vi "Set HW ID.vi"(8 "error in (no error)":errorcluster, 10 "HW ID":dbl, 11 "Controls in":refnum<class "Controls.lvclass">) -> (0 "error out":errorcluster, 3 "Controls out":refnum<class "Controls.lvclass">)   [LabVIEW 2020, in "Controls.lvlib" / "Controls.lvclass"]
uses:
  Controls.lvclass
  Controls.lvclass/Controls.ctl
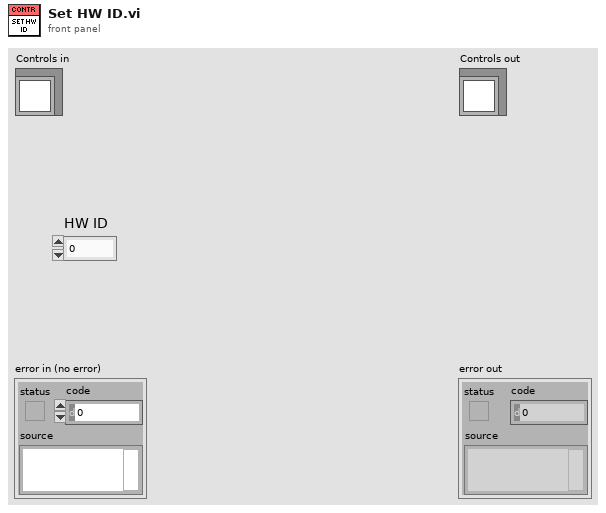
[diagram p1: front panel]
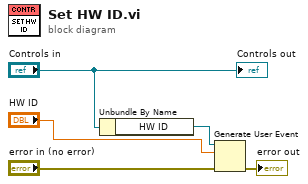
[diagram p0: block diagram]
diagram:
  n1 = Unbundle By Name("Controls in") -> ("HW ID"=w3:refnum<user-event>)
  n2 = Generate User Event(user event=w3, event data cluster="HW ID", error in="error in (no error)") -> (error out=→"error out":errorcluster)  [unwired: 1 in, 1 out]
  "Controls out" <- "Controls in"
